vi "subConvertTargetPathToFilename.vi"(11 "Value in":string) -> (3 "File name":string)   [LabVIEW 2020, in "SolutionBuilder.lvlib"]
uses:
  SolutionBuilder.lvlib
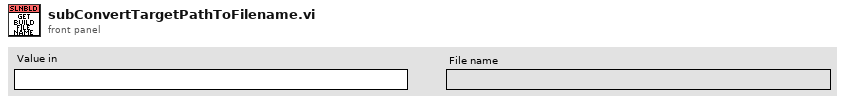
[diagram p1: front panel]
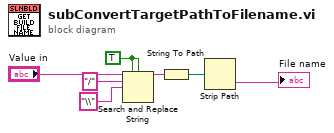
[diagram p0: block diagram]
diagram:
  w5 = TRUE ("replace all? (F)")
  n1 = Search and Replace String(replace all?=w5, case sensitive?=w5, input string="Value in", search string="/", replace string="\\" ("replace string (\"\")")) -> (result string=w4:string)  [unwired: 3 in, 3 out]
  n2 = String To Path(string=w4) -> (path=w1:path)
  n3 = Strip Path(path=w1) -> (name=→"File name":string)  [unwired: 1 out]
